vi "Plot Label TimeToString.vi"(0 "AM/PM":i16, 1 "Time Format":i16, 2 "Time Separator":string=":", 3 "Type (10 = Absolute)":i32, 5 "included seconds":i16, 7 "seconds precision":i16, 9 "m-d-y sequence":i16, 11 "year format":i16, 12 "Date Format":i16, 13 "Date Separator":string="/", 14 "UTC":i16) -> (8 "Format String":string)   [LabVIEW 2020, in "3D Plot.lvclass"]
uses:
  <vilib>/Math Plots/3D Math Plots/3D Plot/3D Plot/3D Plot.lvclass
panel:
  # "0 = AM/PM\n1 = 24 hr"
  # "0 = Custom\n1 = System\n2 = Unused"
  # "0 = nope\n1 = yup"
  # "0 = m-d-y\n1 = d-m-y\n2 = y-m-d"
  # "0 = Local (No DST String)\n1 = UTC (No DST String)\n2 = Local (With DST String)\n3 = UTC (With DST String)"
  # "0 = Custom\n1 = System\n2 = Unused"
  # "0 = no year\n1 = 2 digit\n2 = 4 digit"
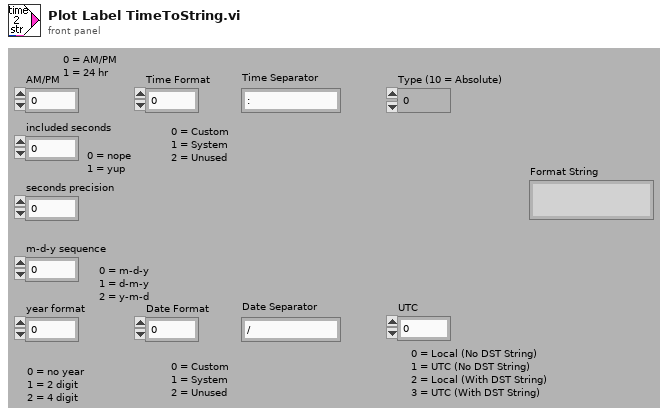
[diagram p1: front panel]
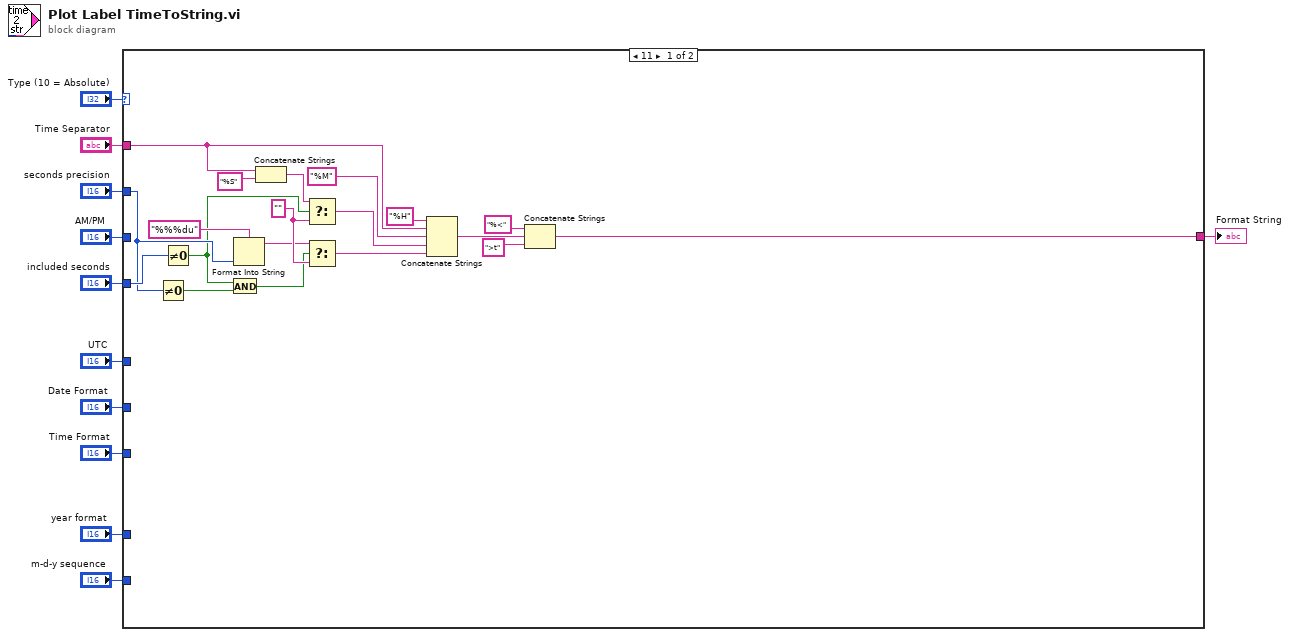
[diagram p0: block diagram]
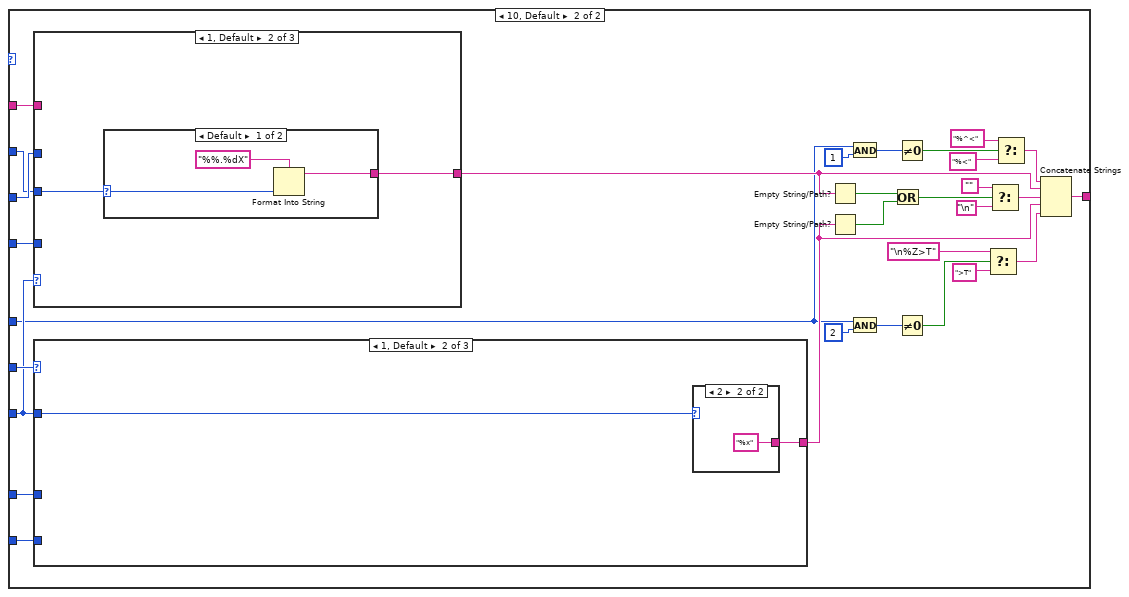
[diagram p2: hidden frame]
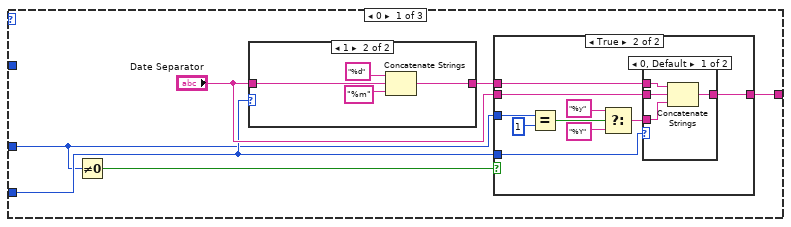
[diagram p3: hidden frame]
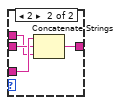
[diagram p5: hidden frame]
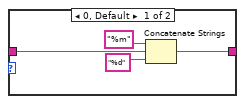
[diagram p6: hidden frame]
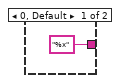
[diagram p7: hidden frame]
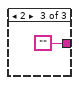
[diagram p8: hidden frame]
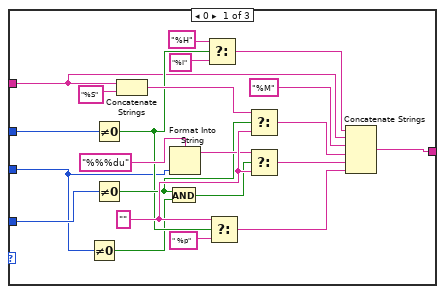
[diagram p9: hidden frame]
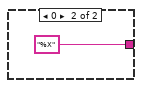
[diagram p10: hidden frame]
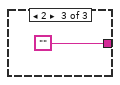
[diagram p11: hidden frame]
diagram:
  n1 = case shown="11" "Type (10 = Absolute)" {
    tunnel: "Date Format" -> [_ w60]
    tunnel: "AM/PM" -> [_ w59]
    tunnel: "included seconds" -> [w30 w58]
    tunnel: "seconds precision" -> [w29 w57]
    tunnel: "m-d-y sequence" -> [_ w56]
    tunnel: "year format" -> [_ w55]
    tunnel: [w26 w54] -> w2
    tunnel: "Time Format" -> [_ w53]
    tunnel: "Time Separator" -> [w13 w52]
    tunnel: "UTC" -> [_ w34]
    frame 11 {
      w21 = ""
      n2 = Not Equal To 0?(x=w29) -> (x != 0?=w15:bool)
      n3 = Not Equal To 0?(x=w30) -> (x != 0?=w16:bool)
      n4 = And(x=w16, y=w15) -> (x .and. y?=w17:bool)
      n5 = Format Into String(format string="%%%du", w29) -> (resulting string=w20:string)  [unwired: 2 in, 1 out]
      n6 = Concatenate Strings(w13, "%S") -> (w24:string)
      n7 = Select(t=w24, s=w16, f=w21) -> (s? t:f=w22:string)
      n8 = Select(t=w20, s=w17, f=w21) -> (s? t:f=w19:string)
      n9 = Concatenate Strings("%H", w13, "%M" ("string"), w22, w19) -> (w28:string)
      n10 = Concatenate Strings("%<" ("string"), w28, ">t") -> (w26:string)
    }
    frame 10, Default {
      n11 = case shown="1, Default" w53 {
        tunnel: [w112 w121 ""] -> w51
        tunnel: w59 -> [w104 _ _]
        tunnel: w58 -> [w102 _ _]
        tunnel: w57 -> [w101 w122 _]
        tunnel: w52 -> [w99 _ _]
        frame 0 {
          w111 = ""
          n12 = Not Equal To 0?(x=w101) -> (x != 0?=w100:bool)
          n13 = Not Equal To 0?(x=w104) -> (x != 0?=w103:bool)
          n14 = Not Equal To 0?(x=w102) -> (x != 0?=w105:bool)
          n15 = Concatenate Strings(w99, "%S") -> (w115:string)
          n16 = And(x=w105, y=w100) -> (x .and. y?=w106:bool)
          n17 = Format Into String(format string="%%%du", w101) -> (resulting string=w110:string)  [unwired: 2 in, 1 out]
          n18 = Select(t="%H", s=w103, f="%I") -> (s? t:f=w117:string)
          n19 = Select(t=w111, s=w103, f=" %p") -> (s? t:f=w107:string)
          n20 = Select(t=w115, s=w105, f=w111) -> (s? t:f=w113:string)
          n21 = Select(t=w110, s=w106, f=w111) -> (s? t:f=w109:string)
          n22 = Concatenate Strings(w117, w99, "%M" ("string"), w113, w109, w107) -> (w112:string)
        }
        frame 1, Default {
          n23 = case shown="Default" w122 {
            selector: w122 -> [w125 _]
            tunnel: [w124 "%X"] -> w121
            frame Default {
              n24 = Format Into String(format string="%%.%dX", w125) -> (resulting string=w124:string)  [unwired: 2 in, 1 out]
            }
            frame 0 {
            }
          }
        }
        frame 2 {
        }
      }
      n25 = case shown="1, Default" w60 {
        tunnel: [w61 w95 ""] -> w45
        tunnel: w56 -> [w64 _ _]
        tunnel: w55 -> [w62 _ _]
        tunnel: w53 -> [_ w94 _]
        frame 0 {
          n26 = Not Equal To 0?(x=w62) -> (x != 0?=w63:bool)
          n27 = case shown="1" w64 {
            tunnel: "Date Separator" -> [w88 w92]
            tunnel: [w86 w90] -> w66
            frame 0, Default {
              n28 = Concatenate Strings("%m", w88, "%d") -> (w86:string)
            }
            frame 1 {
              n29 = Concatenate Strings("%d", w92, "%m") -> (w90:string)
            }
          }
          n30 = case shown="True" w63 {
            tunnel: w66 -> [w67 w77]
            tunnel: "Date Separator" -> [_ w76]
            tunnel: w64 -> [_ w75]
            tunnel: w62 -> [_ w71]
            tunnel: [w67 w68] -> w61
            frame False {
            }
            frame True {
              n31 = Equal?(x=w71, y=i16 1) -> (x = y?=w72:bool)
              n32 = Select(t="%y", s=w72, f="%Y") -> (s? t:f=w69:string)
              n33 = case shown="0, Default" w75 {
                tunnel: w77 -> [w81 w82]
                tunnel: w76 -> [w78 w83]
                tunnel: w69 -> [w80 w84]
                tunnel: [w79 w85] -> w68
                frame 0, Default {
                  n34 = Concatenate Strings(w81, w78, w80) -> (w79:string)
                }
                frame 2 {
                  n35 = Concatenate Strings(w84, w83, w82) -> (w85:string)
                }
              }
            }
          }
        }
        frame 1, Default {
          n36 = case shown="2" w94 {
            tunnel: ["%x" "%x"] -> w95
            frame 0, Default {
            }
            frame 2 {
            }
          }
        }
        frame 2 {
        }
      }
      n37 = Empty String/Path?(string/path=w51) -> (empty?=w50:bool)
      n38 = Empty String/Path?(string/path=w45) -> (empty?=w49:bool)
      n39 = And(x=w34, y=i16 1) -> (x .and. y?=w40:i16)
      n40 = And(x=w34, y=i16 2) -> (x .and. y?=w37:i16)
      n41 = Or(x=w50, y=w49) -> (x .or. y?=w48:bool)
      n42 = Not Equal To 0?(x=w40) -> (x != 0?=w39:bool)
      n43 = Not Equal To 0?(x=w37) -> (x != 0?=w38:bool)
      n44 = Select(t="\n%Z>T", s=w38, f=">T") -> (s? t:f=w32:string)
      n45 = Select(t="", s=w48, f="\n") -> (s? t:f=w44:string)
      n46 = Select(t="%^<", s=w39, f="%<") -> (s? t:f=w33:string)
      n47 = Concatenate Strings(w33, w51, w44, w45, w32) -> (w54:string)
    }
  }
  "Format String" <- w2
